vi "Color-Senser_Read.vi"(6 "觸發數值":dbl=90.0 format="%#_13g", 8 "Error In":errorcluster) -> (0 "Error Out":errorcluster, 3 "觸發?":bool, 5 "當前數值":dbl)   [LabVIEW 2019]
uses:
  <vilib>/myRIO/Instrument Drivers/Onboard IO/AI/AI.lvlib
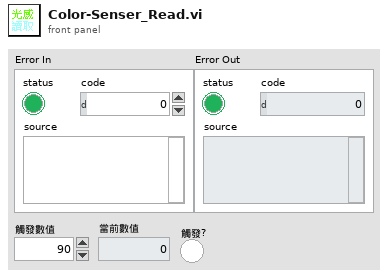
[diagram p1: front panel]
types:
  T1 = typedef "AI.lvlib/AI Reference.ctl" = cluster{"myRIO Reference":T2, "AI Channels List":T6, "AI Scaling Constants List":T8}
  T2 = typedef "myRIO Generic Hardware Reference.ctl" = cluster{"myRIO Model":T3, "myRIO Hardware Reference":T4}
  T3 = typedef "Hardware Version Enum.ctl" = enum16{"Unknown", "myRIO-1900", "myRIO-1950", "roboRIO", "NI ELVIS RIO CM", "ELVIS III"}
  T4 = typedef "myRIO v1.0 Reference.ctl" = cluster{"Generic FPGA Reference":T5, "Allow multiple opens":bool}
  T5 = typedef "Generic FPGA Reference.ctl" = refnum<k20>
  T6 = typedef "AI Channels List.ctl" = T7[]
  T7 = typedef "AI Channels Enum.ctl" = enum16{"Not Connected", "AudioIn/Left", "AudioIn/Right", "C/AI0", "C/AI1", "A/AI0", "A/AI1", "A/AI2", "A/AI3", "A/AI4", "A/AI5", "A/AI6", "A/AI7", "B/AI0", "B/AI1", "B/AI2", "B/AI3", "B/AI4", "B/AI5", "B/AI6", "B/AI7", "AI/AI0", "AI/AI1", "AI/AI2", "AI/AI3", "A/AI0 (DIFF)", "A/AI1 (DIFF)", "A/AI2 (DIFF)", "A/AI3 (DIFF)", "B/AI0 (DIFF)", "B/AI1 (DIFF)", "B/AI2 (DIFF)", "B/AI3 (DIFF)"}
  T8 = typedef "Analog Scaling Constants List.ctl" = T9[]
  T9 = typedef "Analog Scaling Constants.ctl" = cluster{"LSB Weight (Volts)":dbl, "Offset (Volts)":dbl, "Signed?":bool}
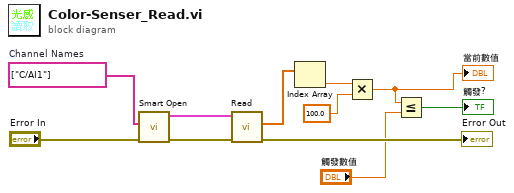
[diagram p0: block diagram]
diagram:
  w11 = tag[] ["C/AI1"]  # Channel Names
  n1 = call <vilib>:"Smart Open.vi"("error in (no error)"="Error In", "Channel Names"=w11) -> ("error out"=w7:errorcluster, "AI Ref Out"=w8:T1)  [unwired: 8 in]
  n2 = call <vilib>:"Read.vi"("error in (no error)"=w7, "AI Ref In"=w8) -> ("error out"=→"Error Out":errorcluster, "Values"=w9:dbl[])  [unwired: 7 in, 1 out]
  n3 = Index Array(array=w9) -> (element=w3:dbl)  [unwired: 1 in]
  n4 = Multiply(x=w3, y=100.0) -> (x*y=w1:dbl)
  "當前數值" <- w1
  n5 = Less Or Equal?(x=w1, y="觸發數值") -> (x <= y?=→"觸發?":bool)
